vi "FileDialog.vi"(8 "Error In":errorcluster, 11 "File Path Control In":path) -> (0 "Error Out":errorcluster, 2 "Valid File Path?":bool, 3 "File Path Control Out":path)   [LabVIEW 2018]
doc: "This VI prompts the user to chose a python file based upon the file location C:\\Users\\ic\\Document\\Scripts\\PV Emulation\\ChromaCurrent.py."
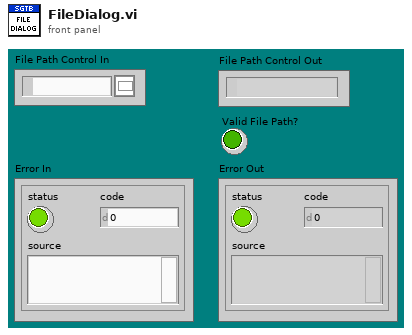
[diagram p1: front panel]
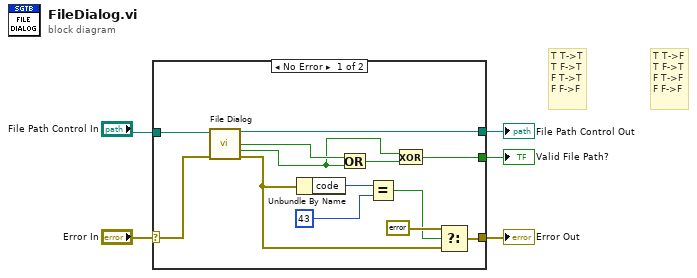
[diagram p0: block diagram]
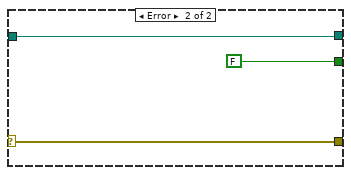
[diagram p2: hidden frame]
diagram:
  # "T T->T\nT F->T\nF T->T\nF F->F"
  # "T T->F\nT F->T\nF T->F\nF F->F"
  n1 = case shown="No Error" "Error In" {
    selector: "Error In" -> [w11 w21]
    tunnel: "File Path Control In" -> [w12 w20]
    tunnel: [w10 w21] -> w4
    tunnel: [w9 w20] -> w2
    tunnel: [w7 FALSE] -> w1
    frame No Error {
      n2 = call "File Dialog"("start path"=w12, "error in"=w11) -> ("selected path"=w9:path, "exists"=w13:bool, "cancelled"=w6:bool, "error out"=w17:errorcluster)  [unwired: 10 in]
      n3 = Unbundle By Name(w17) -> ("code"=w15:i32)
      n4 = Or(x=w13, y=w6) -> (x .or. y?=w8:bool)
      n5 = Equal?(x=w15, y=43 ("code")) -> (x = y?=w14:bool)
      n6 = Exclusive Or(1:w8, 2:w6) -> (0:w7:bool)
      n7 = Select(t=errorcluster {"status"=FALSE, "code"=0, "source"=""} ("error out"), s=w14, f=w17) -> (s? t:f=w10:errorcluster)
    }
    frame Error {
    }
  }
  "Error Out" <- w4
  "File Path Control Out" <- w2
  "Valid File Path?" <- w1
